vi "Initialiser caméra.vi"(8 "entrée d'erreur (pas d'erreur)":errorcluster) -> (0 "sortie d'erreur":errorcluster, 2 "Camera":refnum<class "Camera.lvclass">, 3 "Buffer en sortie":refnum<class "Buffer.lvclass">, 4 "Devices":T1[](array[typedef]), 5 "Pixel Formats":string[](array[string]), 7 "Pixel Format":string)   [LabVIEW 2026]
uses:
  <vilib>/Serenial/G Industrial Camera/g_industrial_cam/Camera/Camera.lvclass
  <vilib>/Serenial/G Industrial Camera/g_industrial_cam/g_industrial_cam.lvlib
  <vilib>/Serenial/G Industrial Camera/g_industrial_cam/Buffer/Buffer.lvclass
  <vilib>/Serenial/G Industrial Camera/g_industrial_cam/Device Enumeration.ctl
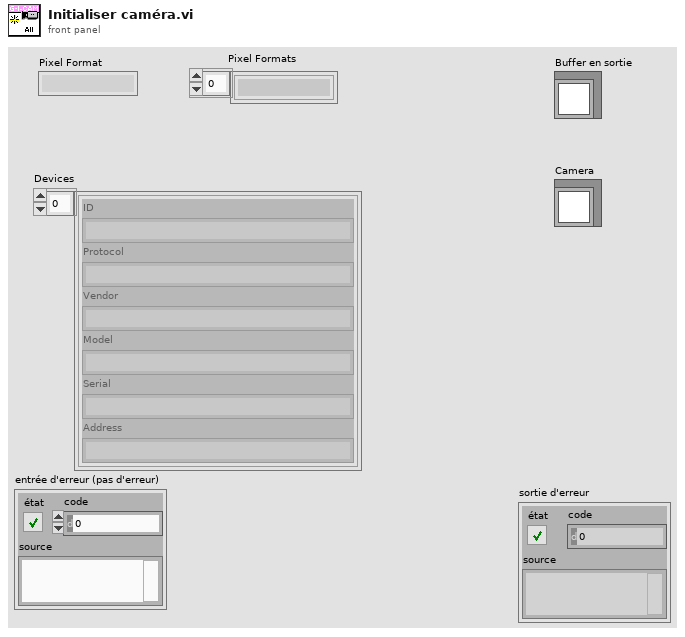
[diagram p1: front panel]
types:
  T1 = typedef "g_industrial_cam.lvlib/Device Enumeration.ctl" = cluster{"ID":string, "Protocol":string, "Vendor":string, "Model":string, "Serial":string, "Address":string}
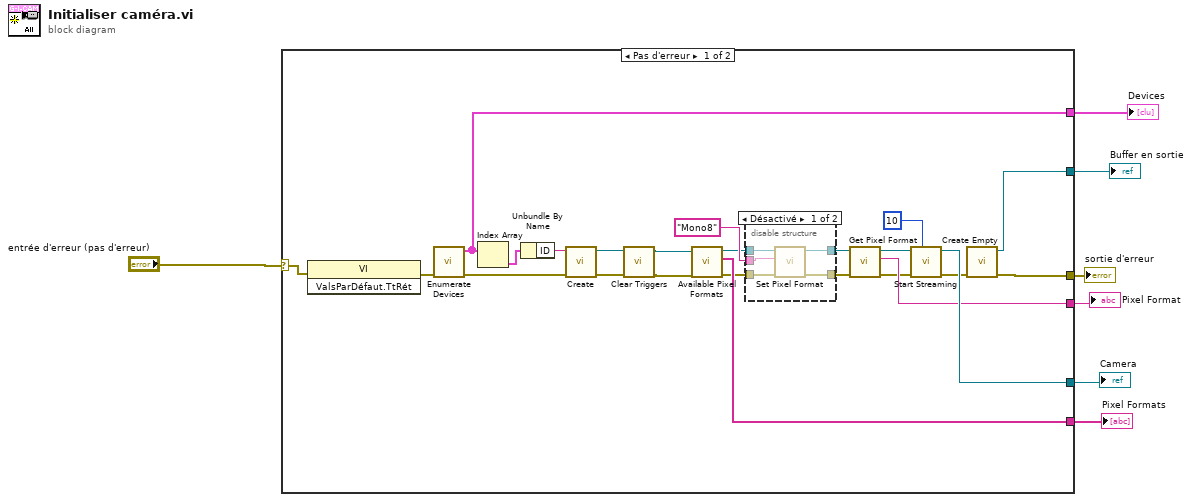
[diagram p0: block diagram]
diagram:
  n1 = case shown="Pas d'erreur" "entrée d'erreur (pas d'erreur)" {
    selector: "entrée d'erreur (pas d'erreur)" -> [w8 w39]
    tunnel: [w31 _] -> w7
    tunnel: [w27 _] -> w6
    tunnel: [w19 _] -> w5
    tunnel: [w17 _] -> w4
    tunnel: [w14 _] -> w3
    tunnel: [w13 w39] -> w2
    frame No Error {
      n2 = invoke class="VI" method="ValsParDéfaut.TtRét"(error in=w8) -> (error out=w24:errorcluster)  [unwired: 2 in, 2 out]
      n3 = call <vilib>:"Enumerate Devices.vi"("error in (no error)"=w24) -> ("error out"=w10:errorcluster, "Devices"=w31:T1[])  [unwired: 9 in]
      n4 = Index Array(array=w31) -> (element=w9:T1)  [unwired: 1 in]
      n5 = Unbundle By Name(w9) -> ("ID"=w11:string)
      n6 = call <vilib>:"Create.vi"("error in (no error)"=w10, "Identifier (ID, IP etc)"=w11) -> ("error out"=w26:errorcluster, "Camera"=w25:refnum<class "Camera.lvclass">)  [unwired: 8 in]
      n7 = call <vilib>:"Clear Triggers.vi"("error in (no error)"=w26, "Camera in"=w25) -> ("error out"=w30:errorcluster, "Camera"=w29:refnum<class "Camera.lvclass">)  [unwired: 8 in]
      n8 = call <vilib>:"Available Pixel Formats.vi"("error in (no error)"=w30, "Camera in"=w29) -> ("error out"=w18:errorcluster, "Pixel Formats"=w19:string[], "Camera"=w21:refnum<class "Camera.lvclass">)  [unwired: 7 in]
      n9 = disable-structure shown="Désactivé" {
        disable-tunnel: w18 -> [w36 w37]
        disable-tunnel: [w35 w37] -> w20
        disable-tunnel: w21 -> [w34 w38]
        disable-tunnel: [w33 w38] -> w22
        disable-tunnel: "Mono8" ("Pixel Format") -> [w32 _]
        frame Disabled {
          n10 = call <vilib>:"Set Pixel Format.vi"("error in (no error)"=w36, "Pixel Format"=w32, "Camera in"=w34) -> ("error out"=w35:errorcluster, "Camera"=w33:refnum<class "Camera.lvclass">)  [unwired: 7 in]
        }
        frame Enabled {
        }
      }
      n11 = call <vilib>:"Get Pixel Format.vi"("error in (no error)"=w20, "Camera in"=w22) -> ("error out"=w15:errorcluster, "Pixel Format"=w17:string, "Camera"=w16:refnum<class "Camera.lvclass">)  [unwired: 7 in]
      n12 = call <vilib>:"Start Streaming.vi"("Additional Buffers (Default: 3)"=u16 10, "error in (no error)"=w15, "Camera in"=w16) -> ("error out"=w12:errorcluster, "Camera"=w27:refnum<class "Camera.lvclass">)  [unwired: 7 in]
      n13 = call <vilib>:"Create Empty.vi"("error in (no error)"=w12) -> ("error out"=w13:errorcluster, "Empty Buffer"=w14:refnum<class "Buffer.lvclass">)  [unwired: 9 in]
    }
    frame Error {
    }
  }
  "Devices" <- w7
  "Pixel Formats" <- w5
  "Camera" <- w6
  "Pixel Format" <- w4
  "Buffer en sortie" <- w3
  "sortie d'erreur" <- w2
